vi "STM32.Relays.vi"(7 "CMD":enum16{"All", "ChanA", "ChanB", "Single"}(ring), 8 "Error In":errorcluster caption="错误输入", 9 "ON/FF":bool, 10 "Para":T1(ring), 11 "VISA资源输入":refnum<visa-resource-name>) -> (0 "Error Out":errorcluster caption="错误输出")   [LabVIEW 2012, in "Lib_UEL.ATE.lvlib" / "STM32-CoreBD.lvlib"]
uses:
  STM32-CoreBD.lvlib
panel:
  out "命令":string
  # "Version History\nV01,2014-4-30, 初始版本."
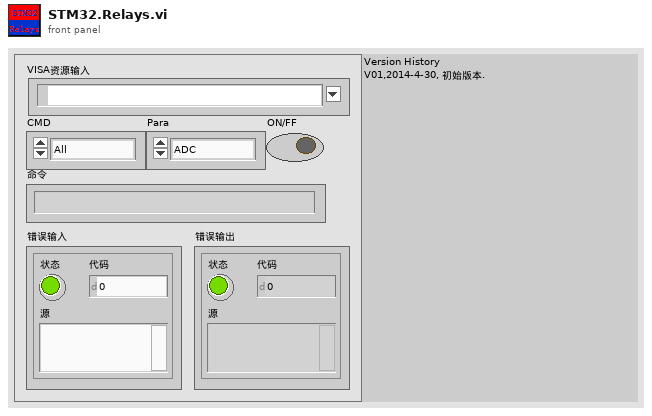
[diagram p1: front panel]
types:
  T1 = enum16{"ADC", "DAC", "RelayA1", "RelayA2", "RelayA3", "RelayA4", "RelayA5", "RelayA6", "RelayA7", "RelayA8", "RelayA9", "RelayA10", "RelayB1", "RelayB2", "RelayB3", "RelayB4", "RelayB5", "RelayB6", "RelayB7", "RelayB8", "RelayB9", "RelayB10"}
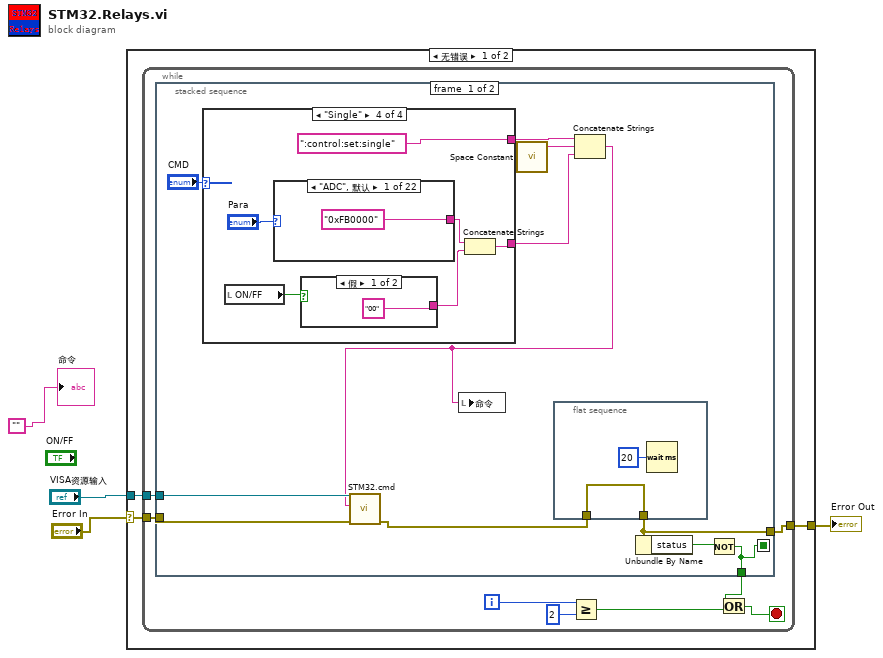
[diagram p0: block diagram]
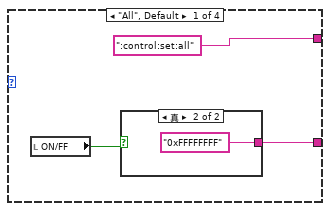
[diagram p2: hidden frame]
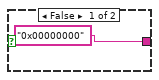
[diagram p3: hidden frame]
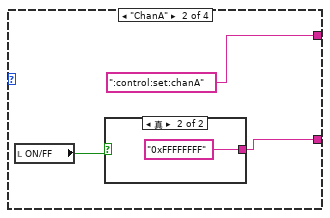
[diagram p4: hidden frame]
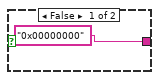
[diagram p5: hidden frame]
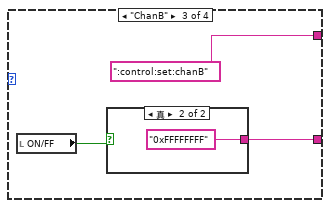
[diagram p6: hidden frame]
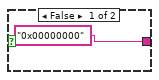
[diagram p7: hidden frame]
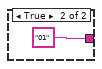
[diagram p8: hidden frame]
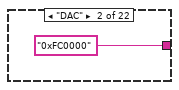
[diagram p9: hidden frame]
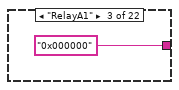
[diagram p10: hidden frame]
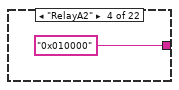
[diagram p11: hidden frame]
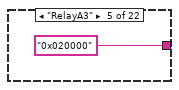
[diagram p12: hidden frame]
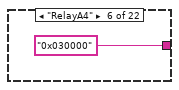
[diagram p13: hidden frame]
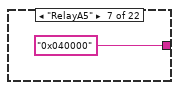
[diagram p14: hidden frame]
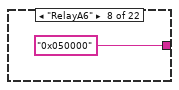
[diagram p15: hidden frame]
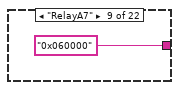
[diagram p16: hidden frame]
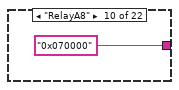
[diagram p17: hidden frame]
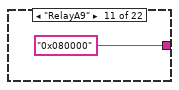
[diagram p18: hidden frame]
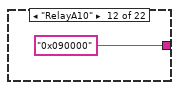
[diagram p19: hidden frame]
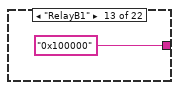
[diagram p20: hidden frame]
diagram:
  n1 = case shown="无错误" "Error In" {
    selector: "Error In" -> [w6 w76]
    tunnel: [w5 w76] -> w4
    tunnel: "VISA资源输入" -> [w7 _]
    frame No Error {
      n2 = while {
        tunnel: w7 -> [w15]
        tunnel: w6 -> [w14]
        tunnel: [w13] -> w5
        i -> [w10]
        stop <- w12 stop-if-true
        n3 = stacked-sequence {
          seq-local: [w17 _] -> [_ w74]
          tunnel: w15 -> [w22 _]
          tunnel: w14 -> [w21 _]
          tunnel: [w19 _] -> w13
          tunnel: [w17 _] -> w11
          frame #0 {
            n4 = case shown="\"Single\"" "CMD" {
              tunnel: [":control:set:all" ("字符串") ":control:set:chanA" ("字符串") ":control:set:chanB" ("字符串") ":control:set:single" ("字符串")] -> w25
              tunnel: [w30 w34 w39 w46] -> w23
              frame "All", Default {
                n5 = local read "ON/FF"() -> (w29:bool)
                n6 = case shown="真" w29 {
                  tunnel: ["0x00000000" ("字符串") "0xFFFFFFFF" ("字符串")] -> w30
                  frame False {
                  }
                  frame True {
                  }
                }
              }
              frame "ChanA" {
                n7 = local read "ON/FF"() -> (w35:bool)
                n8 = case shown="真" w35 {
                  tunnel: ["0x00000000" ("字符串") "0xFFFFFFFF" ("字符串")] -> w34
                  frame False {
                  }
                  frame True {
                  }
                }
              }
              frame "ChanB" {
                n9 = local read "ON/FF"() -> (w40:bool)
                n10 = case shown="真" w40 {
                  tunnel: ["0x00000000" ("字符串") "0xFFFFFFFF" ("字符串")] -> w39
                  frame False {
                  }
                  frame True {
                  }
                }
              }
              frame "Single" {
                n11 = local read "ON/FF"() -> (w47:bool)
                n12 = case shown="\"ADC\", 默认" "Para" {
                  tunnel: ["0xFB0000" ("字符串") "0xFC0000" ("字符串") "0x000000" ("字符串") "0x010000" ("字符串") "0x020000" ("字符串") "0x030000" ("字符串") "0x040000" ("字符串") "0x050000" ("字符串") "0x060000" ("字符串") "0x070000" ("字符串") "0x080000" ("字符串") "0x090000" ("字符串") "0x100000" ("字符串") "0x110000" ("字符串") "0x120000" ("字符串") "0x130000" ("字符串") "0x140000" ("字符串") "0x150000" ("字符串") "0x160000" ("字符串") "0x170000" ("字符串") "0x180000" ("字符串") "0x190000" ("字符串")] -> w45
                  frame "ADC", Default {
                  }
                  frame "DAC" {
                  }
                  frame "RelayA1" {
                  }
                  frame "RelayA2" {
                  }
                  frame "RelayA3" {
                  }
                  frame "RelayA4" {
                  }
                  frame "RelayA5" {
                  }
                  frame "RelayA6" {
                  }
                  frame "RelayA7" {
                  }
                  frame "RelayA8" {
                  }
                  frame "RelayA9" {
                  }
                  frame "RelayA10" {
                  }
                  frame "RelayB1" {
                  }
                  frame "RelayB2" {
                  }
                  frame "RelayB3" {
                  }
                  frame "RelayB4" {
                  }
                  frame "RelayB5" {
                  }
                  frame "RelayB6" {
                  }
                  frame "RelayB7" {
                  }
                  frame "RelayB8" {
                  }
                  frame "RelayB9" {
                  }
                  frame "RelayB10" {
                  }
                }
                n13 = case shown="假" w47 {
                  tunnel: ["00" ("字符串") "01" ("字符串")] -> w44
                  frame False {
                  }
                  frame True {
                  }
                }
                n14 = Concatenate Strings(w45, w44) -> (w46:string)
              }
            }
            n15 = call <vilib>:"Space Constant.vi"() -> ("String"=w24:string)
            n16 = flat-sequence {
              tunnel: [w28] -> w19
              tunnel: w20 -> [w28]
              frame #0 {
                n17 = Wait (ms)(milliseconds to wait=u32 20 ("等待时间（毫秒）")) -> ()  [unwired: 1 out]
              }
            }
            n18 = Concatenate Strings(w25, w24, w23) -> (w16:string)
            n19 = call "STM32.cmd.vi"("Error In"=w21, "命令"=w16, "VISA资源输入"=w22) -> ("Error Out"=w20:errorcluster)  [unwired: 5 in, 3 out]
            n20 = local write "命令"(w16) -> ()
            n21 = Unbundle By Name(w19) -> ("status"=w18:bool)
            n22 = Not(x=w18) -> (.not. x?=w17:bool)
          }
          frame #1 {
            n23 = case shown="假" w74 {
              frame False {
                n24 = Wait (ms)(milliseconds to wait=u32 500 ("等待时间（毫秒）")) -> ()  [unwired: 1 out]
              }
              frame True {
              }
            }
          }
        }
        n25 = Greater Or Equal?(x=w10, y=2) -> (x >= y?=w8:bool)
        n26 = Or(x=w11, y=w8) -> (x .or. y?=w12:bool)
      }
    }
    frame Error {
    }
  }
  "Error Out" <- w4
  "命令" <- ""
